vi "VPI Set PWM Pulse.vi"(7 "pPulse":string, 8 "error in (no error)":errorcluster, 9 "ChannelMask":u8, 10 "DevIndex":i32, 11 "DevType":i32) -> (0 "error out":errorcluster, 3 "function return":i32)   [LabVIEW 2012, in "ControlPWM.lvlib"]
doc: "int WINAPI VPI_SetPWMPulse(int DevType, int DevIndex, unsigned char ChannelMask,unsigned char *pPulse);"
uses:
  ControlPWM.lvlib
  Ginkgo_Driver.dll
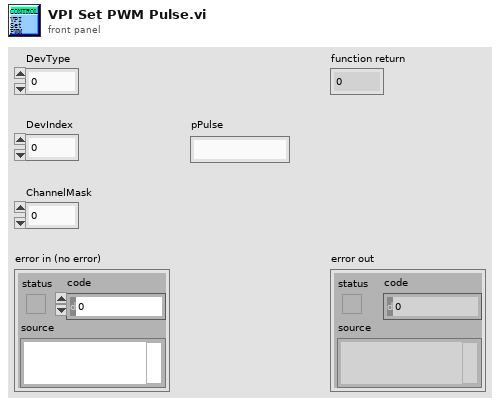
[diagram p1: front panel]
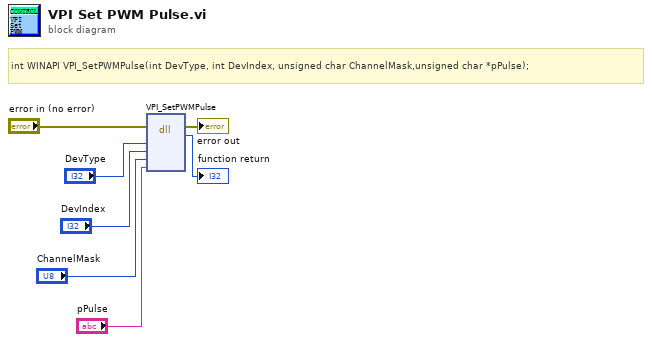
[diagram p0: block diagram]
diagram:
  # "int\tWINAPI VPI_SetPWMPulse(int DevType, int DevIndex, unsigned char ChannelMask,unsigned char *pPulse);"
  n1 = dll-call lib="E:/Project/vt_ginkgo/truck/Ginkgo Driver/vs2010/Ginkgo_USB-I2C_API_v2.0.3.0/lib/labview_32bit/ControlPWM/Ginkgo_Driver.*" fn="VPI_SetPWMPulse"(error in="error in (no error)", "DevType"="DevType", "DevIndex"="DevIndex", "ChannelMask"="ChannelMask", "pPulse"="pPulse") -> (error out=→"error out":errorcluster, →"function return":i32)  [unwired: 6 in, 1 out]
